vi "ErrorLogRead.vi"(8 "error in (no error)":errorcluster) -> (0 "error out":errorcluster)   [LabVIEW 2019]
uses:
  <vilib>/Utility/file.llb/Read Delimited Spreadsheet (string).vi
panel:
  out "all rows":string[][](array[string])
  out "讀到的Error紀錄":errorcluster[](array[cluster])
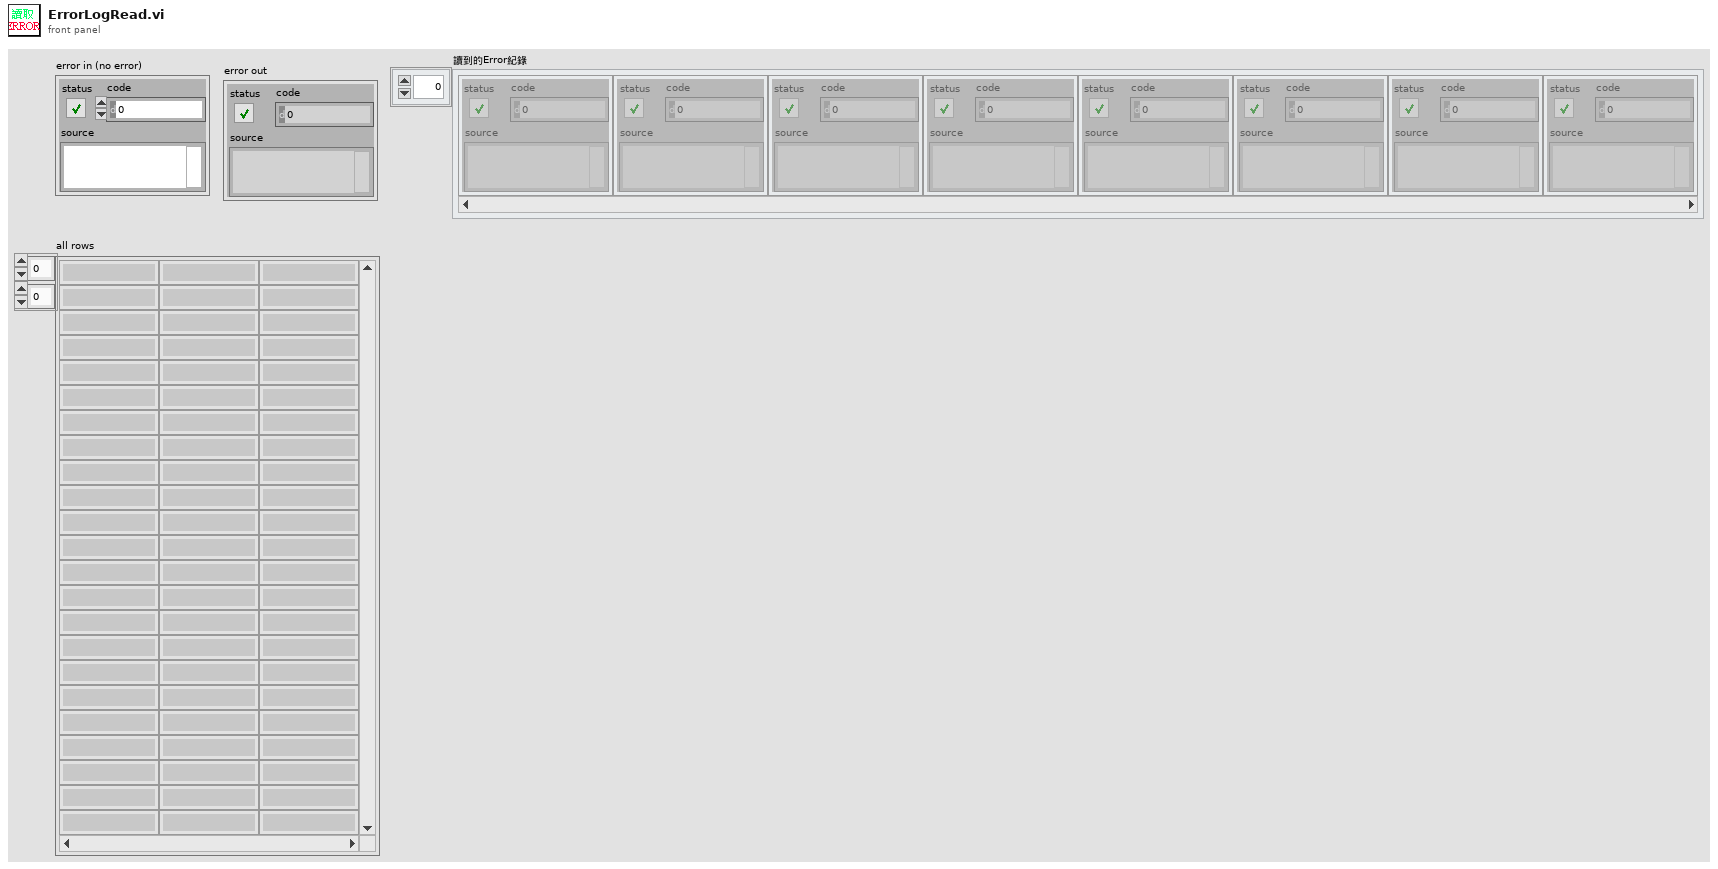
[diagram p1: front panel]
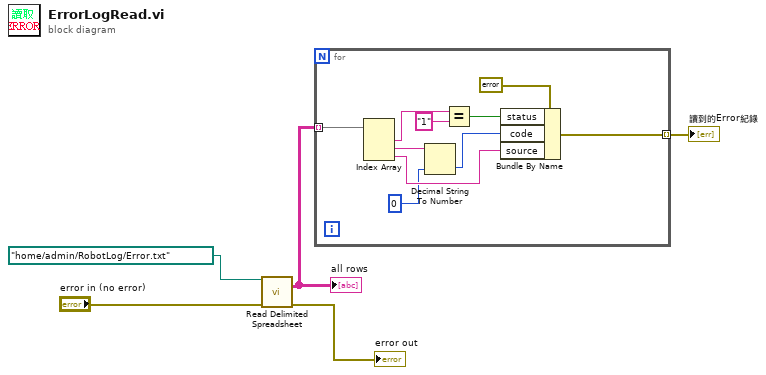
[diagram p0: block diagram]
diagram:
  n1 = call-poly <vilib>:"Read Delimited Spreadsheet.vi"("file path (dialog if empty)"=path "/home/admin/RobotLog/Error.txt", "error in (no error)"="error in (no error)") -> ("all rows"=w2:string[][], "error out"=→"error out":errorcluster)  [unwired: 8 in, 4 out]
  "all rows" <- w2
  n2 = for {
    tunnel: w2 -> [w7] mode=indexing
    tunnel: [w6] -> w1 mode=indexing
    n3 = Index Array(array=w7) -> (element #1=w14:string, element #2=w11:string, element #3=w10:string)  [unwired: 3 in]
    n4 = Decimal String To Number(string=w11, default (0L)=0 ("code")) -> (number=w8:i32)  [unwired: 1 in, 1 out]
    n5 = Equal?(x=w14, y="1") -> (x = y?=w12:bool)
    n6 = Bundle By Name(cluster=errorcluster {"status"=FALSE, "code"=0, "source"=""} ("讀到的Error紀錄 2"), "status"=w12, "code"=w8, "source"=w10) -> (w6:errorcluster)
  }
  "讀到的Error紀錄" <- w1
